vi "GetWindowRect.vi"(8 "error in (no error)":errorcluster, 11 "hWnd (NULL)":T2) -> (0 "error out":errorcluster, 2 "Rect":T1, 3 "dup hWnd":T2)   [LabVIEW 2011]
doc: "GetWindowRect\nThe GetWindowRect function retrieves the dimensions of the bounding rectangle of the specified window. The dimensions are given in screen coordinates that are relative to the upper-left corner of the screen. \n\nBOOL GetWindowRect(\n HWND hWnd, // handle to window\n LPRECT lpRect // address of structure for window coordinates\n);\n \nParameters\nhWnd \nHandle to the window. \nlpRect \nPointer to aRECT structure that receives the screen coordinates of the upper-left and lower-right corners of the window. \nReturn Values\nIf the function succeeds, the return value is nonzero.\n\nIf the function fails, the return value is zero. To get extended error information, callGetLastError."
uses:
  hWnd.ctl
  user32.dll
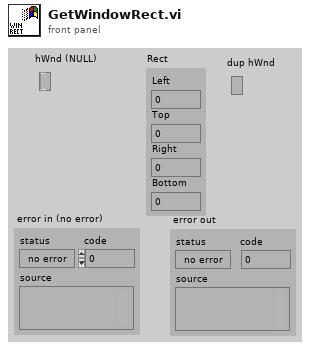
[diagram p1: front panel]
types:
  T1 = cluster{"Left":i32, "Top":i32, "Right":i32, "Bottom":i32}
  T2 = typedef "hWnd.ctl" = refnum<k1>
  T3 = cluster{"RECT[0]":i32, "RECT[1]":i32, "RECT[2]":i32, "RECT[3]":i32}
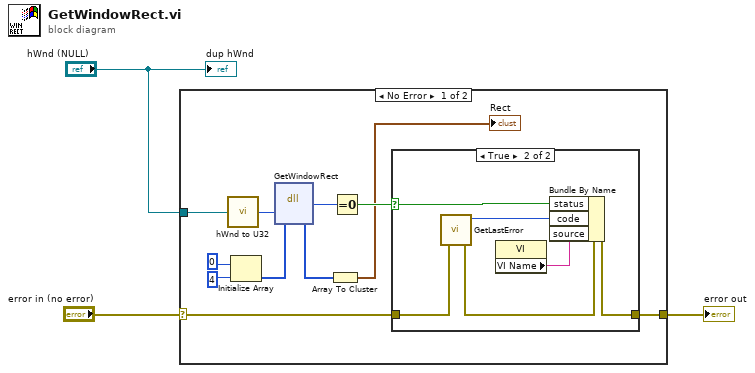
[diagram p0: block diagram]
diagram:
  n1 = case shown="No Error" "error in (no error)" {
    selector: "error in (no error)" -> [w8 w22]
    tunnel: [w9 w22] -> w3
    tunnel: "hWnd (NULL)" -> [w5 _]
    frame No Error {
      n2 = call "hWnd to U32.vi"("hWnd"=w5) -> ("hWnd"=w6:u32)  [unwired: 4 out]
      n3 = Initialize Array(0, 4) -> (w12:i32[])
      n4 = dll-call lib="User32.dll" fn="GetWindowRect"("hWnd"=w6, "RECT"=w12) -> ("Return Value"=w10:i32, "RECT"=w11:i32[])  [unwired: 4 in, 2 out]
      n5 = Array To Cluster(array=w11) -> (cluster=→"Rect":T3)
      n6 = Equal To 0?(x=w10) -> (x = 0?=w7:bool)
      n7 = case shown="True" w7 {
        selector: w7 -> [_ w16]
        tunnel: w8 -> [w15 w20]
        tunnel: [w15 w21] -> w9
        frame False {
        }
        frame True {
          n8 = call "GetLastError.vi"("error in (no error)"=w20) -> ("error out"=w19:errorcluster, "CODE"=w18:i32)  [unwired: 5 out]
          n9 = property class="VI"() -> ("VI Name"=w17:string)  [unwired: 2 in, 2 out]
          n10 = Bundle By Name(cluster=w19, "status"=w16, "code"=w18, "source"=w17) -> (w21:errorcluster)
        }
      }
    }
    frame Error {
    }
  }
  "error out" <- w3
  "dup hWnd" <- "hWnd (NULL)"
